vi "Pane Relief Main UI.vi"(6 "Stopped Event":refnum<user-event>, 8 "Error In":errorcluster, 9 "Splitter Colors":T1={"Normal"=13816530, "Mouse-over"=0, "Selected"=9868950, "Selected Mouse-over"=9868950}, 10 "Pane Colors":T1={"Normal"=13816530, "Mouse-over"=0, "Selected"=9868950, "Selected Mouse-over"=9868950}, 11 "QD Launch VI Ref":refnum<vi>) -> (0 "Error Out":errorcluster, 3 "Pane Relief Main UI out":refnum<class "Pane Relief Main UI.lvclass">)   [LabVIEW 2017, in "Pane Relief Main UI.lvlib" / "Pane Relief Main UI.lvclass"]
uses:
  Pane Relief Main UI.lvclass
  Typedefs/Selection Colors--Cluster.ctl
  Pane Relief Main UI.lvclass/Pane Relief Main UI.ctl
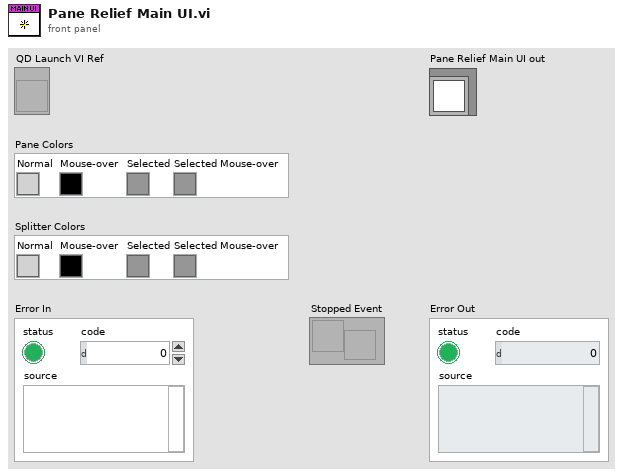
[diagram p1: front panel]
types:
  T1 = typedef "Selection Colors--Cluster.ctl" = cluster{"Normal":u32, "Mouse-over":u32, "Selected":u32, "Selected Mouse-over":u32}
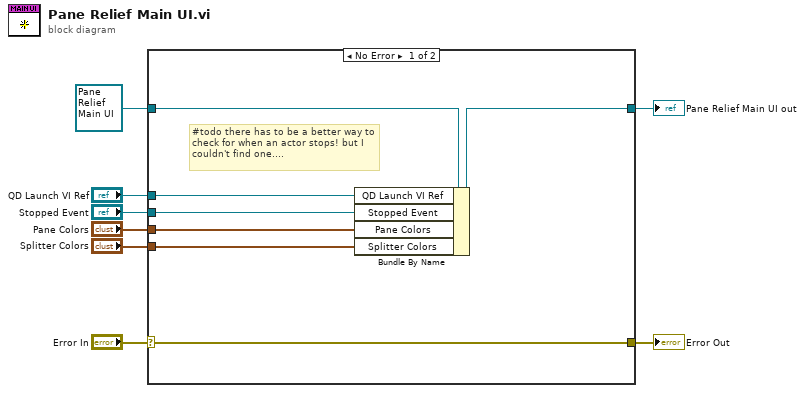
[diagram p0: block diagram]
diagram:
  n1 = case shown="No Error" "Error In" {
    selector: "Error In" -> [w15 w17]
    tunnel: [w15 w17] -> w6
    tunnel: [w14 w16] -> w8
    tunnel: refnum<class "Pane Relief Main UI.lvclass"> refnum ("Pane Relief Main UI in") -> [w13 w16]
    tunnel: "QD Launch VI Ref" -> [w12 _]
    tunnel: "Stopped Event" -> [w11 _]
    tunnel: "Pane Colors" -> [w10 _]
    tunnel: "Splitter Colors" -> [w9 _]
    frame No Error {
      # "#todo there has to be a better way to check for when an actor stops! but I couldn't find one...."
      n2 = Bundle By Name(cluster=w13, "QD Launch VI Ref"=w12, "Stopped Event"=w11, "Pane Colors"=w10, "Splitter Colors"=w9) -> (w14:refnum<class "Pane Relief Main UI.lvclass">)
    }
    frame Error {
    }
  }
  "Pane Relief Main UI out" <- w8
  "Error Out" <- w6
